vi "Convert Relative Move to String.vi"(8 "Relative Object Name":string, 9 "Relative Movement Type":T1, 10 "Y":i32, 11 "X":i32) -> (3 "String":string)   [LabVIEW 2020, in "MacroAssert.lvlib" / "Mouse Action.lvclass"]
uses:
  Mouse Action.lvclass
  Relative Movement Type.ctl
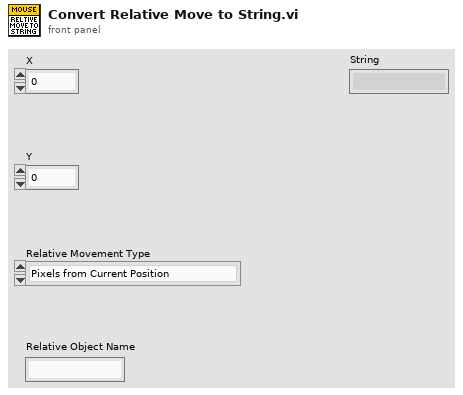
[diagram p1: front panel]
types:
  T1 = typedef "MacroAssert.lvlib/Mouse Action.lvclass/Relative Movement Type.ctl" = enum16{"Pixels from Current Position", "Pixels from Top-Left of Control", "Pixels from Top-Left of Window", "Percentage from Top-Left of Control", "Percentage from Top-Left of Window", "Percentage from Top-Left of Screen"}
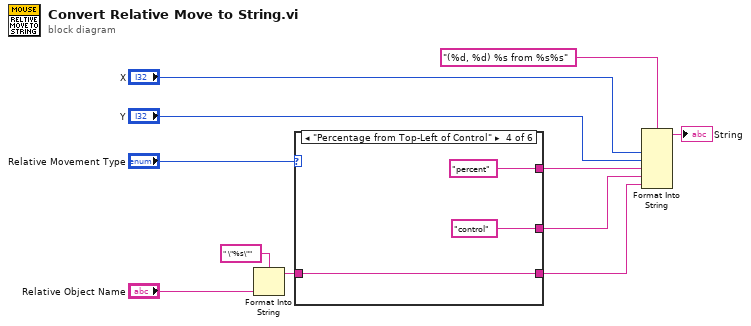
[diagram p0: block diagram]
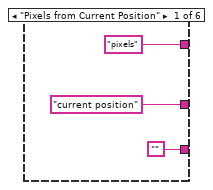
[diagram p2: hidden frame]
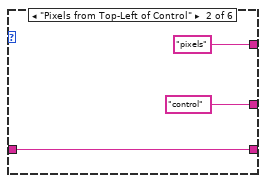
[diagram p3: hidden frame]
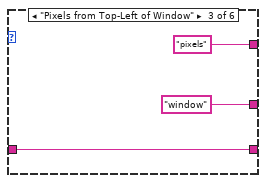
[diagram p4: hidden frame]
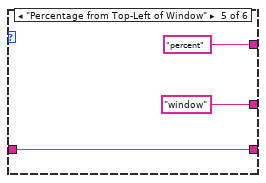
[diagram p5: hidden frame]
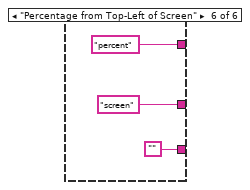
[diagram p6: hidden frame]
diagram:
  n1 = Format Into String(format string=" \"%s\"", "Relative Object Name") -> (resulting string=w1:string)  [unwired: 2 in, 1 out]
  n2 = case shown="\"Percentage from Top-Left of Control\"" "Relative Movement Type" {
    tunnel: ["pixels" ("format string") "pixels" ("format string") "pixels" ("format string") "percent" ("format string") "percent" ("format string") "percent" ("format string")] -> w7
    tunnel: ["current position" ("format string") "control" ("format string") "window" ("format string") "control" ("format string") "window" ("format string") "screen" ("format string")] -> w8
    tunnel: w1 -> [_ w15 w18 w21 w24 _]
    tunnel: ["" ("Relative Object Name") w15 w18 w21 w24 "" ("Relative Object Name")] -> w9
    frame "Pixels from Current Position" {
    }
    frame "Pixels from Top-Left of Control" {
    }
    frame "Pixels from Top-Left of Window" {
    }
    frame "Percentage from Top-Left of Control" {
    }
    frame "Percentage from Top-Left of Window" {
    }
    frame "Percentage from Top-Left of Screen" {
    }
  }
  n3 = Format Into String(format string="(%d, %d) %s from %s%s", "X", "Y", w7, w8, w9) -> (resulting string=→"String":string)  [unwired: 2 in, 1 out]
